vi "Parallel For Loop Iteration Order.vi"() -> ()   [LabVIEW 2023]
doc: "This VI shows how the iterations of a Parallel For Loop can be interleaved when executed on a machine with multiple cores or processors."
panel:
  out "Actual Instances":i32
  in  "Parallel Instances":i32=1 min=1
  out "Chart":i32(graph)
  # "Overview: Demonstrates the use of a Parallel For Loop to execute multiple iterations of the same For Loop in parallel.\nInstructions:\n1. Run the VI. With a single parallel instance, all iterations of the For Loop happen in order.\n2. Increase the value of the Parallel Instances control.\n3. Run the VI again. Observe that multiple iterations now execute at the same time. If the specified number of Parallel Instances exceeds the number of processors on your machine, you will no longer see a difference in the appearance of the graph."
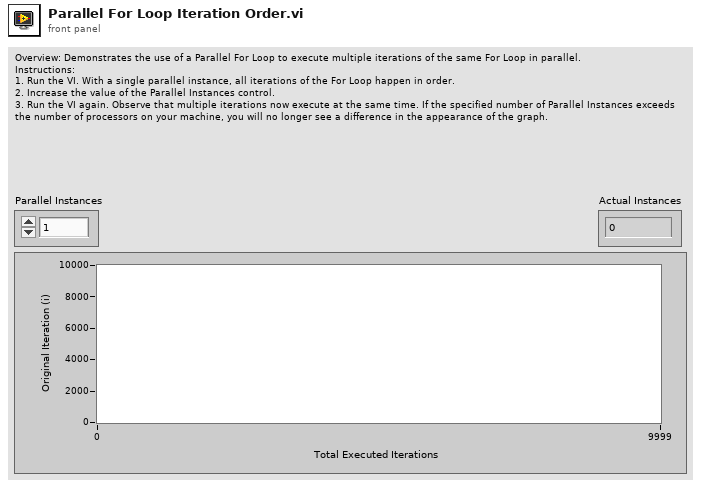
[diagram p1: front panel]
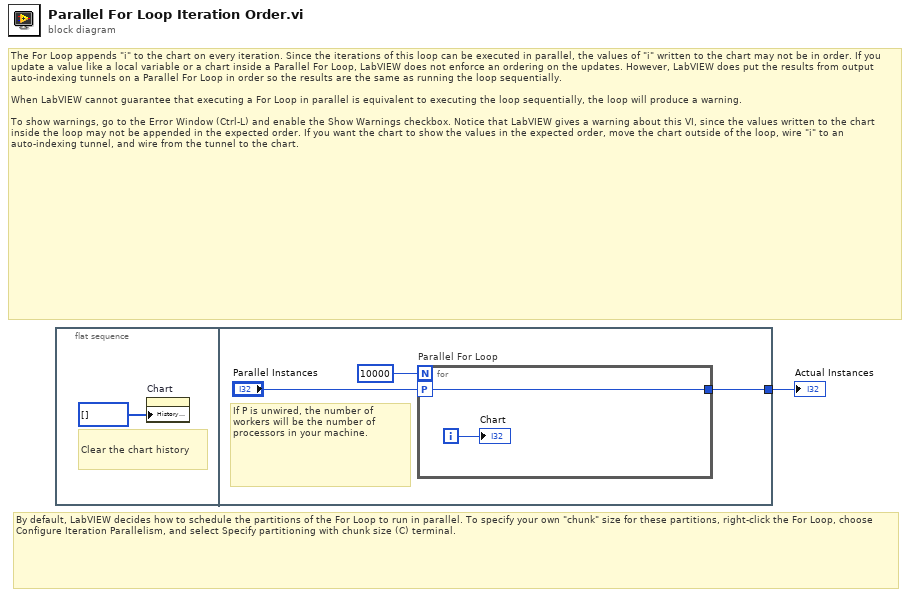
[diagram p0: block diagram]
diagram:
  # "By default, LabVIEW decides how to schedule the partitions of the For Loop to run in parallel. To specify your own \"chunk\" size for these partitions, right-click the For Loop, choose Configure Iteration Parallelism, and select Specify partitioning with chunk size (C) terminal."
  # "The For Loop appends \"i\" to the chart on every iteration. Since the iterations of this loop can be executed in parallel, the values of \"i\" written to the chart may not be in order. If you update a value like a local variable or a chart inside a Parallel For Loop, LabVIEW does not enforce an ordering on the updates. However, LabVIEW does put the results from output auto-indexing tunnels on a Parallel For Loop in order so the results are the same as running the loop sequentially.\n\nWhen LabVIEW cannot guarantee that executing a For Loop in parallel is equivalent to executing the loop sequentially, the loop will produce a warning.\n\nTo show warnings, go to the Error Window (Ctrl-L) and enable the Show Warnings checkbox. Notice that LabVIEW gives a warning about this VI, since the values written to the chart inside the loop may not be appended in the expected order. If you want the chart to show the values in the expected order, move the chart outside of the loop, wire \"i\" to an auto-indexing tunnel, and wire from the tunnel to the chart."
  n1 = flat-sequence {
    tunnel: [w3] -> w1
    frame #0 {
      # "Clear the chart history"
      n2 = property on="Chart" class="WFChart (strict)"("History Data"=i32[] []) -> ()  [unwired: 2 in, 2 out]
    }
    frame #1 {
      # "If P is unwired, the number of workers will be the number of processors in your machine."
      n3 = for "Parallel For Loop" {
        N: 10000 ("# of Iterations") -> [_]
        workers-P: "Parallel Instances" -> [w6]
        tunnel: [w6] -> w3
        i -> [w7]
        "Chart" <- w7
      }
    }
  }
  "Actual Instances" <- w1
